vi "Engine Offset (Plugin).vi"(8 "error in (no error)":errorcluster, 11 "Plugin Configuration in":T1={"name"="", "components"=[], "cycle timing"={"priority"=0, "decimation"=1, "offset"=0}, "Transfer Groups"=[], "thread count"=1, "buffer converter settings"=[], "transceiver settings"=[]} {"Transfer Groups"."Transfers"."channels"."dst buffer offset" format="%d bytes"; "Transfer Groups"."Transfers"."channels"."src buffer offset" format="%d bytes"}) -> (0 "error out":errorcluster, 2 "engine offset":u64, 3 "Plugin Configuration out":T1={"name"="", "components"=[], "cycle timing"={"priority"=0, "decimation"=1, "offset"=0}, "Transfer Groups"=[], "thread count"=1, "buffer converter settings"=[], "transceiver settings"=[]} {"Transfer Groups"."Transfers"."channels"."dst buffer offset" format="%d bytes"; "Transfer Groups"."Transfers"."channels"."src buffer offset" format="%d bytes"})   [LabVIEW 2017, in "DSF Core.lvlib"]
uses:
  DSF Core.lvlib
  Controls/DSF Engine Plugin Configuration.ctl
  Controls/DSF Timing Info.ctl
  Controls/DSF Engine Transfer Group Configuration.ctl
  Controls/DSF Direction.ctl
  Controls/DSF Engine Transfer Configuration.ctl
  Controls/DSF Byte Order.ctl
  Controls/DSF Engine Channel Configuration.ctl
  Controls/DSF Data Type.ctl
  Controls/DSF Settings Info.ctl
  Engine Offset (Transfer).vi
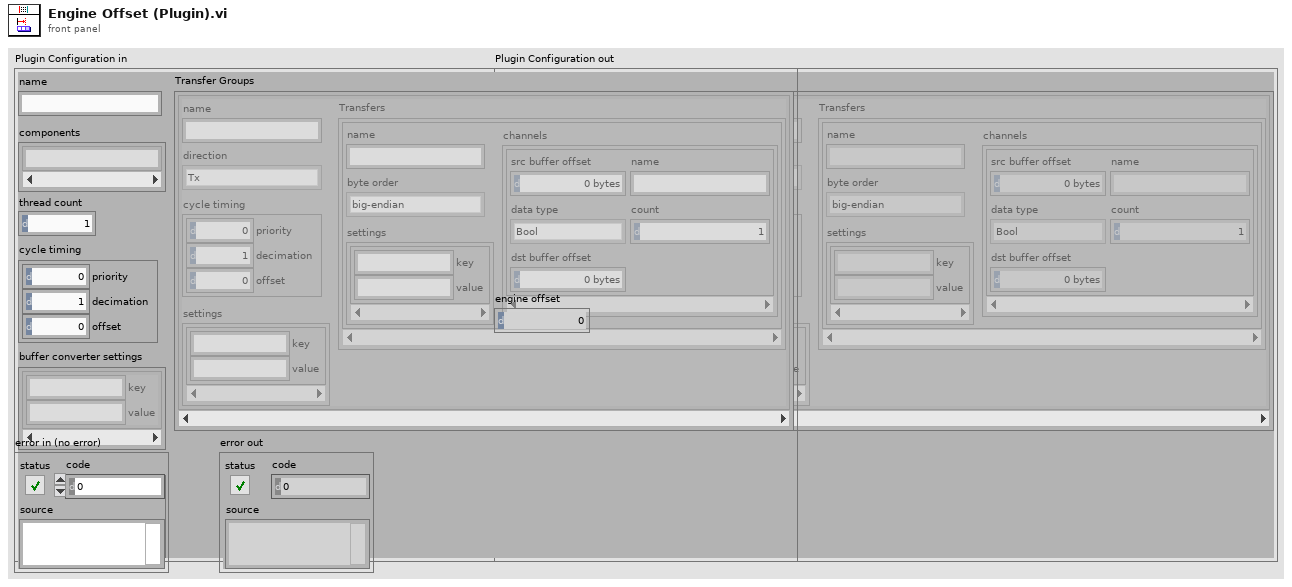
[diagram p1: front panel]
types:
  T1 = typedef "DSF Core.lvlib/DSF Engine Plugin Configuration.ctl" = cluster{"name":string, "components":string[], "cycle timing":T2, "Transfer Groups":T3[], "thread count":i32, "buffer converter settings":T9, "transceiver settings":T9}
  T2 = typedef "DSF Core.lvlib/DSF Timing Info.ctl" = cluster{"priority":u64, "decimation":u64, "offset":u64}
  T3 = typedef "DSF Core.lvlib/DSF Engine Transfer Group Configuration.ctl" = cluster{"name":string, "direction":T4, "cycle timing":T2, "Transfers":T5[], "settings":T9}
  T4 = typedef "DSF Core.lvlib/DSF Direction.ctl" = enum8{"Tx", "Rx"}
  T5 = typedef "DSF Core.lvlib/DSF Engine Transfer Configuration.ctl" = cluster{"name":string, "byte order":T6, "channels":T7[], "settings":T9}
  T6 = typedef "DSF Core.lvlib/DSF Byte Order.ctl" = enum8{"big-endian", "little-endian"}
  T7 = typedef "DSF Core.lvlib/DSF Engine Channel Configuration.ctl" = cluster{"src buffer offset":u64, "name":string, "data type":T8, "count":u64, "dst buffer offset":u64}
  T8 = typedef "DSF Core.lvlib/DSF Data Type.ctl" = enum8{"Bool", "SGL", "DBL", "I8", "I16", "I32", "I64", "U8", "U16", "U32", "U64"}
  T9 = typedef "DSF Core.lvlib/DSF Settings Info.ctl" = cluster{"key":string, "value":string}[]
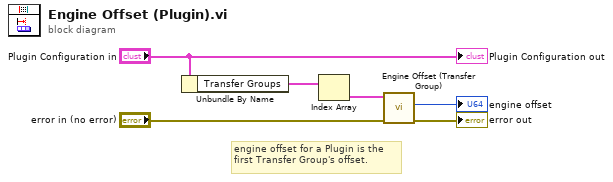
[diagram p0: block diagram]
diagram:
  # "engine offset for a Plugin is the first Transfer Group's offset."
  n1 = Unbundle By Name("Plugin Configuration in") -> ("Transfer Groups"=w5:T3[])
  n2 = Index Array(array=w5) -> (element=w4:T3)  [unwired: 1 in]
  n3 = call "Engine Offset (Transfer Group).vi"("error in (no error)"="error in (no error)", "Transfer Group Configuration in"=w4) -> ("error out"=→"error out":errorcluster, "engine offset"=→"engine offset":u64)  [unwired: 7 in, 1 out]
  "Plugin Configuration out" <- "Plugin Configuration in"
